vi "Dereference Face.vi"(8 "error in (no error)":errorcluster, 11 "face in":i64) -> (0 "error out":errorcluster, 2 "Face":T1, 3 "face out":i64)   [LabVIEW 2023, in "Freetype Drawer.lvlib"]
uses:
  Freetype Drawer.lvlib
  Face.ctl
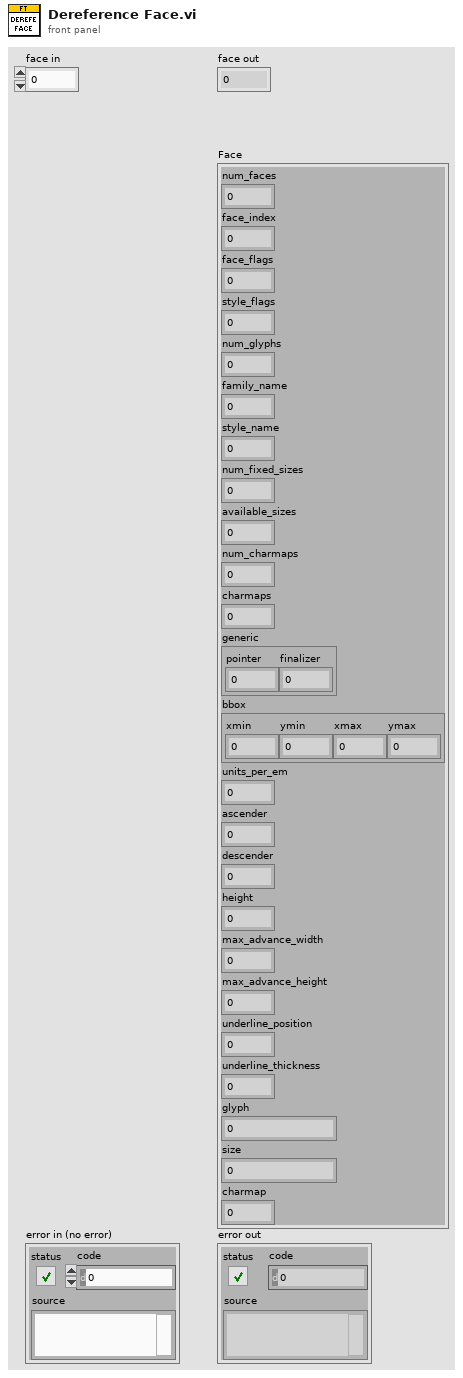
[diagram p1: front panel]
types:
  T1 = typedef "Freetype Drawer.lvlib/Face.ctl" = cluster{"num_faces":i32, "face_index":i32, "face_flags":i32, "style_flags":i32, "num_glyphs":i32, "family_name":i64, "style_name":i64, "num_fixed_sizes":i32, "available_sizes":i64, "num_charmaps":i32, "charmaps":i64, "generic":cluster{"pointer":i64, "finalizer":i64}, "bbox":cluster{"xmin":i32, "ymin":i32, "xmax":i32, "ymax":i32}, "units_per_em":u16, "ascender":i16, "descender":i16, "height":i16, "max_advance_width":i16, "max_advance_height":i16, "underline_position":i16, "underline_thickness":i16, "glyph":i64, "size":i64, "charmap":i64}
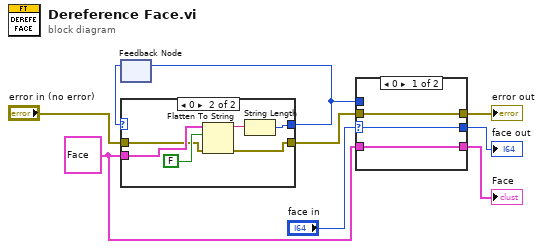
[diagram p0: block diagram]
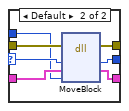
[diagram p2: hidden frame]
diagram:
  w7 = T1 {"num_faces"=0, "face_index"=0, "face_flags"=0, "style_flags"=0, "num_glyphs"=0, "family_name"=0, "style_name"=0, "num_fixed_sizes"=0, "available_sizes"=0, "num_charmaps"=0, "charmaps"=0, "generic"={"pointer"=0, "finalizer"=0}, "bbox"={"xmin"=0, "ymin"=0, "xmax"=0, "ymax"=0}, "units_per_em"=0, "ascender"=0, "descender"=0, "height"=0, "max_advance_width"=0, "max_advance_height"=0, "underline_position"=0, "underline_thickness"=0, "glyph"=0, "size"=0, "charmap"=0} ("Face")
  n1 = feedback #1() -> (w1:i32)  [unwired: 1 in]
  n2 = case shown="0" w1 {
    selector: w1 -> [w11 _]
    tunnel: w7 -> [_ w15]
    tunnel: "error in (no error)" -> [w10 w14]
    tunnel: [w10 w13] -> w3
    tunnel: [w11 w12] -> w2
    frame Default {
    }
    frame 0 {
      n3 = Flatten To String(anything=w15, prepend array or string size? (T)=FALSE, error in (no error)=w14) -> (data string=w17:string, error out=w13:errorcluster)  [unwired: 1 in, 1 out]
      n4 = String Length(string=w17) -> (length=w12:i32)
    }
  }
  n5 = feedback-in #1(w2) -> ()
  n6 = case shown="0" "face in" {
    selector: "face in" -> [w19 w23]
    tunnel: [w20 w27] -> w9
    tunnel: [w18 w26] -> w8
    tunnel: w7 -> [w18 w25]
    tunnel: [w19 w24] -> w6
    tunnel: w3 -> [w20 w22]
    tunnel: w2 -> [_ w21]
    frame 0 {
    }
    frame Default {
      n7 = dll-call lib="LabVIEW" fn="MoveBlock"(error in=w22, "in"=w23, "out"=w25, "size"=w21) -> (error out=w27:errorcluster, "in"=w24:i64, "out"=w26:T1)  [unwired: 4 in, 1 out]
    }
  }
  "error out" <- w9
  "Face" <- w8
  "face out" <- w6
